vi "dfd_Dolph Chebyshev Window.vi"(9 "r [dB]":dbl format="%.2f", 11 "x(t)":dbl[](array[numeric])) -> (0 "error":i32, 3 "Dolph-Chebyshev":dbl[](array[numeric]) format="%.2f")   [LabVIEW 2017, in "NI_DigFilter_Design.lvlib"]
uses:
  <vilib>/addons/Digital Filter Design/NI_DigFilter_Design.lvlib
  <vilib>/Analysis/1siggen.llb/Ramp Pattern by Samples.vi
  <vilib>/addons/Digital Filter Design/NI_DigFilterLicensed.lvlib
  <vilib>/Analysis/NI_AALBase.lvlib
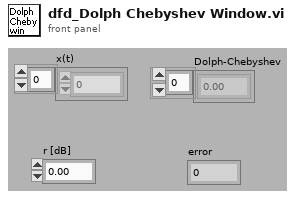
[diagram p1: front panel]
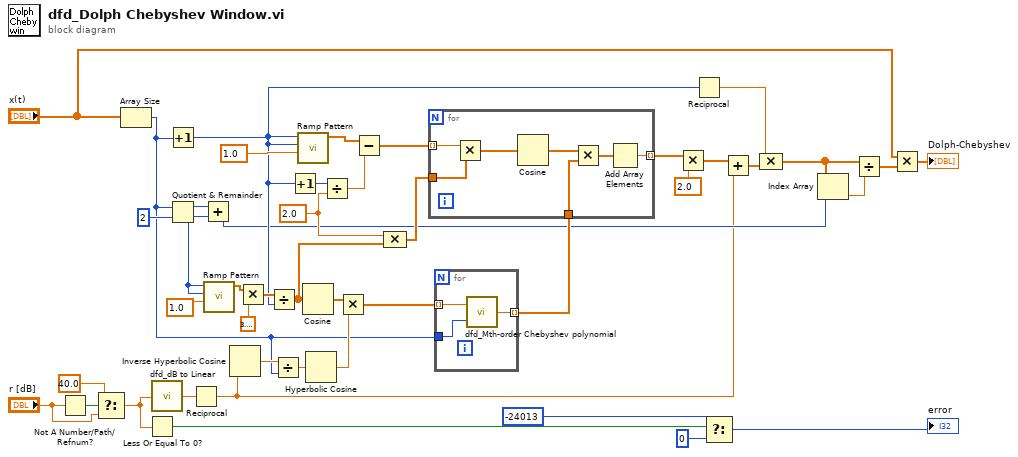
[diagram p0: block diagram]
diagram:
  w35 = 2.0 ("y")
  n1 = Not A Number/Path/Refnum?(number/path/refnum="r [dB]") -> (NaN/Path/Refnum?=w4:bool)
  n2 = Select(t=40.0, s=w4, f="r [dB]") -> (s? t:f=w2:dbl)
  n3 = Array Size(array="x(t)") -> (size(s)=w12:i32)
  n4 = Less Or Equal To 0?(x=w2) -> (x <= 0?=w8:bool)
  n5 = call <vilib>:"dfd_dB to Linear.vi"("dB value"=w2) -> ("linear value"=w13:dbl)  [unwired: 1 in]
  n6 = Increment(x=w12) -> (x+1=w29:i32)
  n7 = Quotient & Remainder(x=w12, y=2) -> (x-y*floor(x/y)=w24:i32, floor(x/y)=w25:i32)
  n8 = Reciprocal(x=w13) -> (1/x=w19:dbl)
  n9 = Add(x=w24, y=w25) -> (x+y=w22:i32)
  n10 = call-poly <vilib>:"Ramp Pattern.vi"("start"=1.0, "end"=w25, "samples"=w25) -> ("Ramp Pattern"=w43:dbl[])  [unwired: 7 in, 1 out]
  n11 = Inverse Hyperbolic Cosine(1:w19) -> (0:w21:dbl)
  n12 = Multiply(x=w43, y=3.141592653589793) -> (x*y=w42:dbl[])
  n13 = Divide(x=w42, y=w29) -> (x/y=w36:dbl[])
  n14 = Divide(x=w21, y=w12) -> (x/y=w20:dbl)
  n15 = Increment(x=w29) -> (x+1=w37:i32)
  n16 = call-poly <vilib>:"Ramp Pattern.vi"("start"=1.0, "end"=w29, "samples"=w29) -> ("Ramp Pattern"=w38:dbl[])  [unwired: 7 in, 1 out]
  n17 = Cosine(x=w36) -> (cos(x)=w41:dbl[])
  n18 = Hyperbolic Cosine(1:w20) -> (0:w18:dbl)
  n19 = Divide(x=w37, y=w35) -> (x/y=w23:dbl)
  n20 = Multiply(x=w41, y=w18) -> (x*y=w40:dbl[])
  n21 = Subtract(x=w38, y=w23) -> (x-y=w34:dbl[])
  n22 = Compound Arithmetic op=MULTIPLY(w35, w36) -> (w33:dbl[])
  n23 = for {
    tunnel: w40 -> [w47] mode=indexing
    tunnel: w12 -> [w46]
    tunnel: [w45] -> w32 mode=indexing
    n24 = call <vilib>:"dfd_Mth-order Chebyshev polynomial.vi"("M"=w46, "x"=w47) -> ("CM(x)"=w45:dbl)
  }
  n25 = for {
    tunnel: w34 -> [w54] mode=indexing
    tunnel: w33 -> [w53]
    tunnel: w32 -> [w50]
    tunnel: [w48] -> w31 mode=indexing
    n26 = Multiply(x=w54, y=w53) -> (x*y=w52:dbl[])
    n27 = Cosine(x=w52) -> (cos(x)=w51:dbl[])
    n28 = Multiply(x=w51, y=w50) -> (x*y=w49:dbl[])
    n29 = Add Array Elements(numeric array=w49) -> (sum=w48:dbl)
  }
  n30 = Multiply(x=w31, y=2.0) -> (x*y=w30:dbl[])
  n31 = Reciprocal(x=w29) -> (1/x=w28:dbl)
  n32 = Select(t=-24013 ("ERR_R4DOLPH_LE_ZERO"), s=w8, f=0) -> (s? t:f=→"error":i32)
  n33 = Add(x=w30, y=w19) -> (x+y=w15:dbl[])
  n34 = Compound Arithmetic op=MULTIPLY(w28, w15) -> (w14:dbl[])
  n35 = Index Array(array=w14, index=w22) -> (element=w26:dbl)
  n36 = Divide(x=w14, y=w26) -> (x/y=w11:dbl[])
  n37 = Multiply(x="x(t)", y=w11) -> (x*y=→"Dolph-Chebyshev":dbl[])
